vi "Single Item Save Dark Current.vi"(10 "String":string, 11 "Numeric":dbl) -> ()   [LabVIEW 2020]
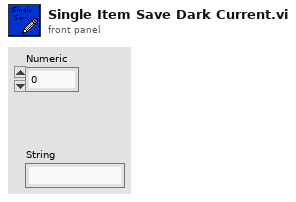
[diagram p1: front panel]
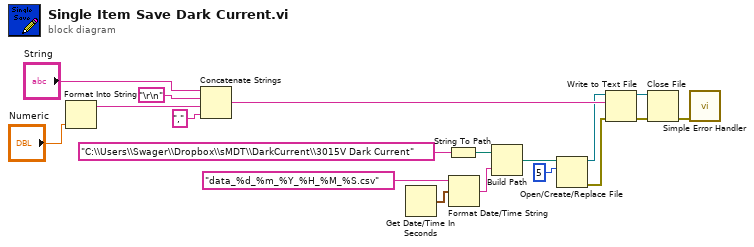
[diagram p0: block diagram]
diagram:
  n1 = Format Into String("Numeric") -> (resulting string=w16:string)  [unwired: 3 in, 1 out]
  n2 = Concatenate Strings("String", "\r\n", w16, ",") -> (w13:string)
  n3 = Get Date/Time In Seconds() -> (seconds since 1Jan1904=w3:timestamp)
  n4 = String To Path(string="C:\\Users\\Swager\\Dropbox\\sMDT\\DarkCurrent\\3015V Dark Current") -> (path=w4:path)
  n5 = Format Date/Time String(time format string (%c)="data_%d_%m_%Y_%H_%M_%S.csv", seconds (now)=w3) -> (date/time string=w2:string)  [unwired: 1 in]
  n6 = Build Path(base path=w4, name or relative path=w2) -> (appended path=w6:path)
  n7 = Open/Create/Replace File(file path (use dialog)=w6, operation (0:open)=5) -> (refnum out=w7:refnum<file>, error out=w8:errorcluster)  [unwired: 4 in, 1 out]
  n8 = Write to Text File(file (use dialog)=w7, text=w13, error in=w8) -> (refnum out=w9:refnum<file>, error out=w10:errorcluster)  [unwired: 1 in, 1 out]
  n9 = Close File(refnum=w9, error in=w10) -> (error out=w11:errorcluster)  [unwired: 1 out]
  n10 = call <vilib>:"Simple Error Handler.vi"("error in (no error)"=w11) -> ()  [unwired: 4 in, 5 out]
